vi "Read Key Value Path.vi"(7 "Section Name":string, 8 "error in (no error)":errorcluster, 9 "Default":path, 10 "Key Name":string, 11 "Ini-File in":refnum<class "Ini-File.lvclass">) -> (0 "error out":errorcluster, 1 "Value":path, 2 "found":bool, 3 "Ini-File out":refnum<class "Ini-File.lvclass">)   [LabVIEW 2016, in "Configuration.lvlib" / "Ini-File.lvclass"]
doc: "Read path key value."
uses:
  Ini-File.lvclass
  Ini-File.lvclass/Ini-File.ctl
  <vilib>/Utility/config.llb/Read Key (Path).vi
  <vilib>/Utility/config.llb/NI_LVConfig.lvlib
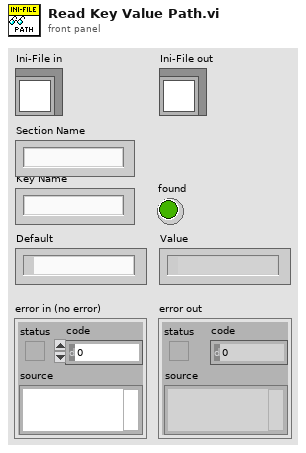
[diagram p1: front panel]
types:
  T1 = typedef "NI_LVConfig.lvlib/Config Data RefNum.ctl" = refnum<k1>
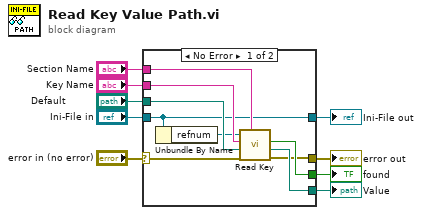
[diagram p0: block diagram]
diagram:
  n1 = case shown="No Error" "error in (no error)" {
    selector: "error in (no error)" -> [w12 w20]
    tunnel: "Section Name" -> [w18 _]
    tunnel: "Key Name" -> [w17 _]
    tunnel: "Default" -> [w16 _]
    tunnel: [w14 _] -> w5
    tunnel: [w15 _] -> w6
    tunnel: [w13 w20] -> w7
    tunnel: "Ini-File in" -> [w11 w19]
    tunnel: [w11 w19] -> w8
    frame No Error {
      n2 = Unbundle By Name(w11) -> ("refnum"=w10:T1)
      n3 = call-poly <vilib>:"Read Key.vi"("section"=w18, "error in (no error)"=w12, "default value"=w16, "key"=w17, "refnum"=w10) -> ("error out"=w13:errorcluster, "value"=w14:path, "found?"=w15:bool)  [unwired: 3 in, 1 out]
    }
    frame Error {
    }
  }
  "error out" <- w7
  "Ini-File out" <- w8
  "Value" <- w5
  "found" <- w6
